vi "Plot_Channels_TF.vi"() -> (5 "Plug in titles":string[](array[string]), 7 "Plug in values":string[](array[string]))   [LabVIEW 2011]
uses:
  Controls/XY_Plot_Cluster.ctl
  Globals/Meas_global.vi
panel:
  out "Stats Array":string[][](array[string])
  in  "Run Spectra":bool=TRUE
  in  "Run Stats":bool=TRUE
  in  "Time delay":dbl
  in  "Save plot":bool
  in  "Save Plot":bool
  out "XY Graph 2":cluster{"Time (ms)":dbl[], "Eng Values":dbl[]}[](graph)
  out "Stats out":T1
  out "Size 2":i32
  out "Size 1":i32
  out "Size 0":i32
  in  "interp. method":i32(ring) items=["nearest", "linear", "spline", "cubic Hermite", "Lagrange"]
  in  "index 2":i32=3
  out "XY Graph":cluster{"Time (ms)":dbl[], "Eng Values":dbl[]}[](graph)
  in  "index 1":i32=1
  in  "index 0":i32
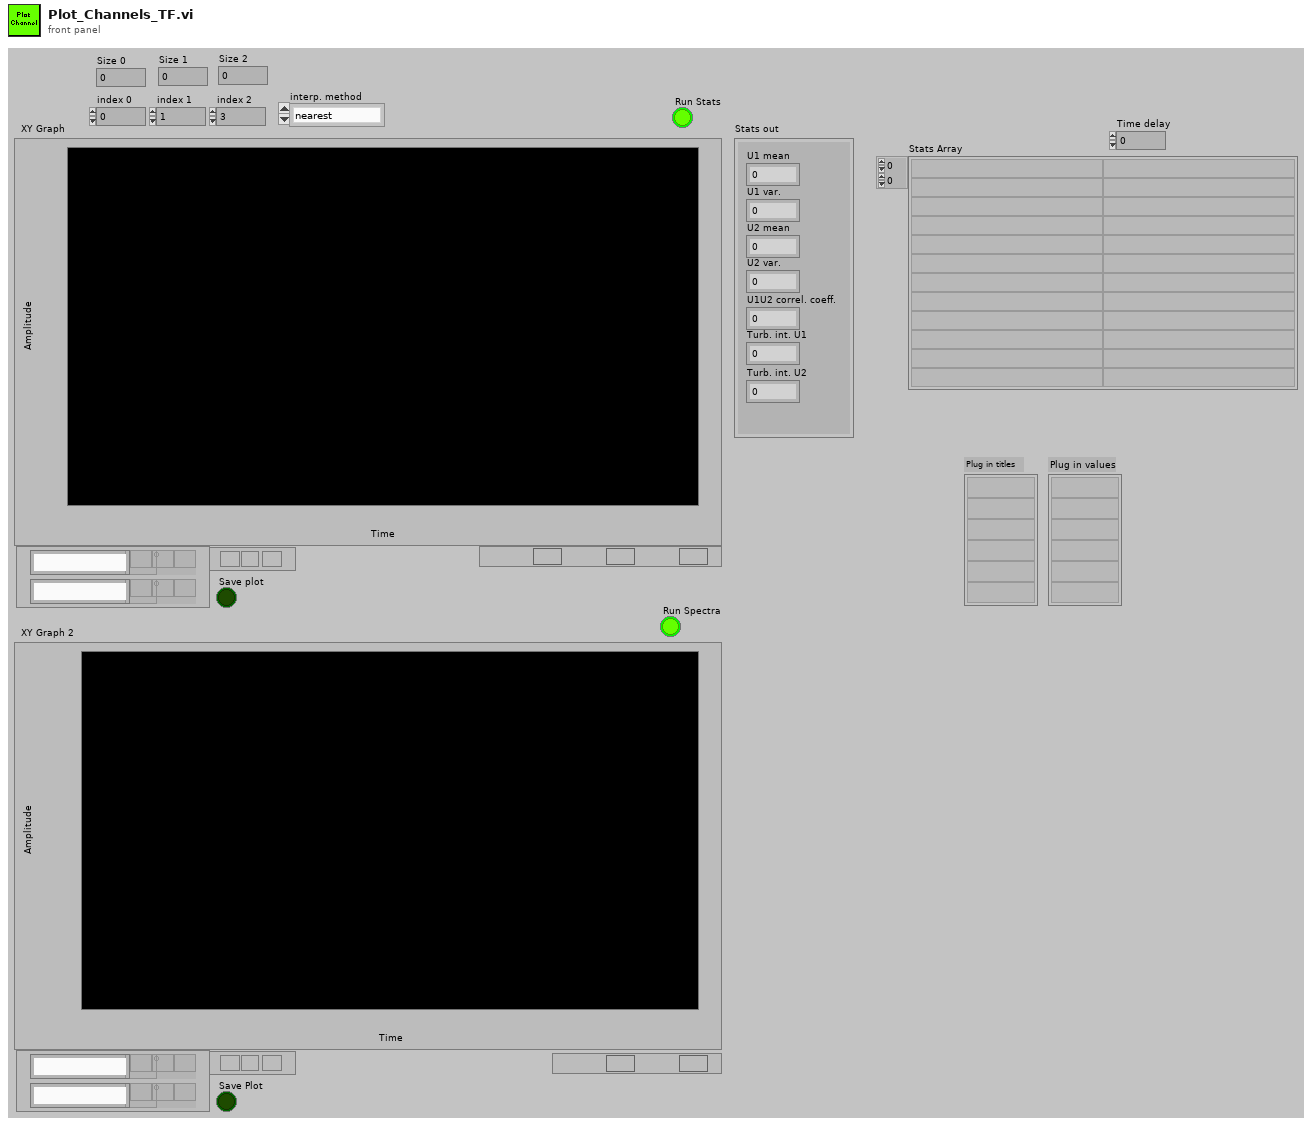
[diagram p1: front panel]
types:
  T1 = cluster{"U1 mean":dbl, "U1 var.":dbl, "U2 mean":dbl, "U2 var.":dbl, "U1U2 correl. coeff.":dbl, "Turb. int. U1":dbl, "Turb. int. U2":dbl}
  T2 = typedef "Analysis_info_cluster.ctl" = cluster{"Colour":u32, "Inst type":T3, "Inst name":string, "Symbol":string, "Code name":string, "Extra Info":string, "Inst Array":T4, "Index":i32, "Voltage Index":i32, "Extra Titles":string[], "Extra Values":string[], "Eng Values":dbl[], "Time (ms)":dbl[], "TT / Voltage":dbl[], "U":dbl, "u^2":dbl, "u^3":dbl, "u^4":dbl, "Skew_u":dbl, "Kurt_u":dbl, "Mean % Err":dbl, "% u'/U":dbl, "X":dbl, "Y":dbl, "Z":dbl}
  T3 = typedef "Inst_type.ctl" = enum16{"Propeller anemometer", "Raw voltage", "Pressure Transducer", "Pitot-static tube", "Preston tube", "Hot wire", "Cross wire 1", "Cross wire 2", "Generic Linear", "Generic Polynomial", "Generic BackPoly", "Fast FID", "Thermocouple", "Cold wire", "Pulsed Wire", "LDA Vel", "LDA Tran time", "LDA Arr time"}
  T4 = typedef "Instrument_Array.ctl" = enum16{"PWA", "LDA", "Analogue"}
  T5 = typedef "XY_Plot_Cluster.ctl" = cluster{"First Name":string, "Second Name":string, "X axis name":string, "Y axis name":string, "X array":dbl[], "Y array":dbl[]}
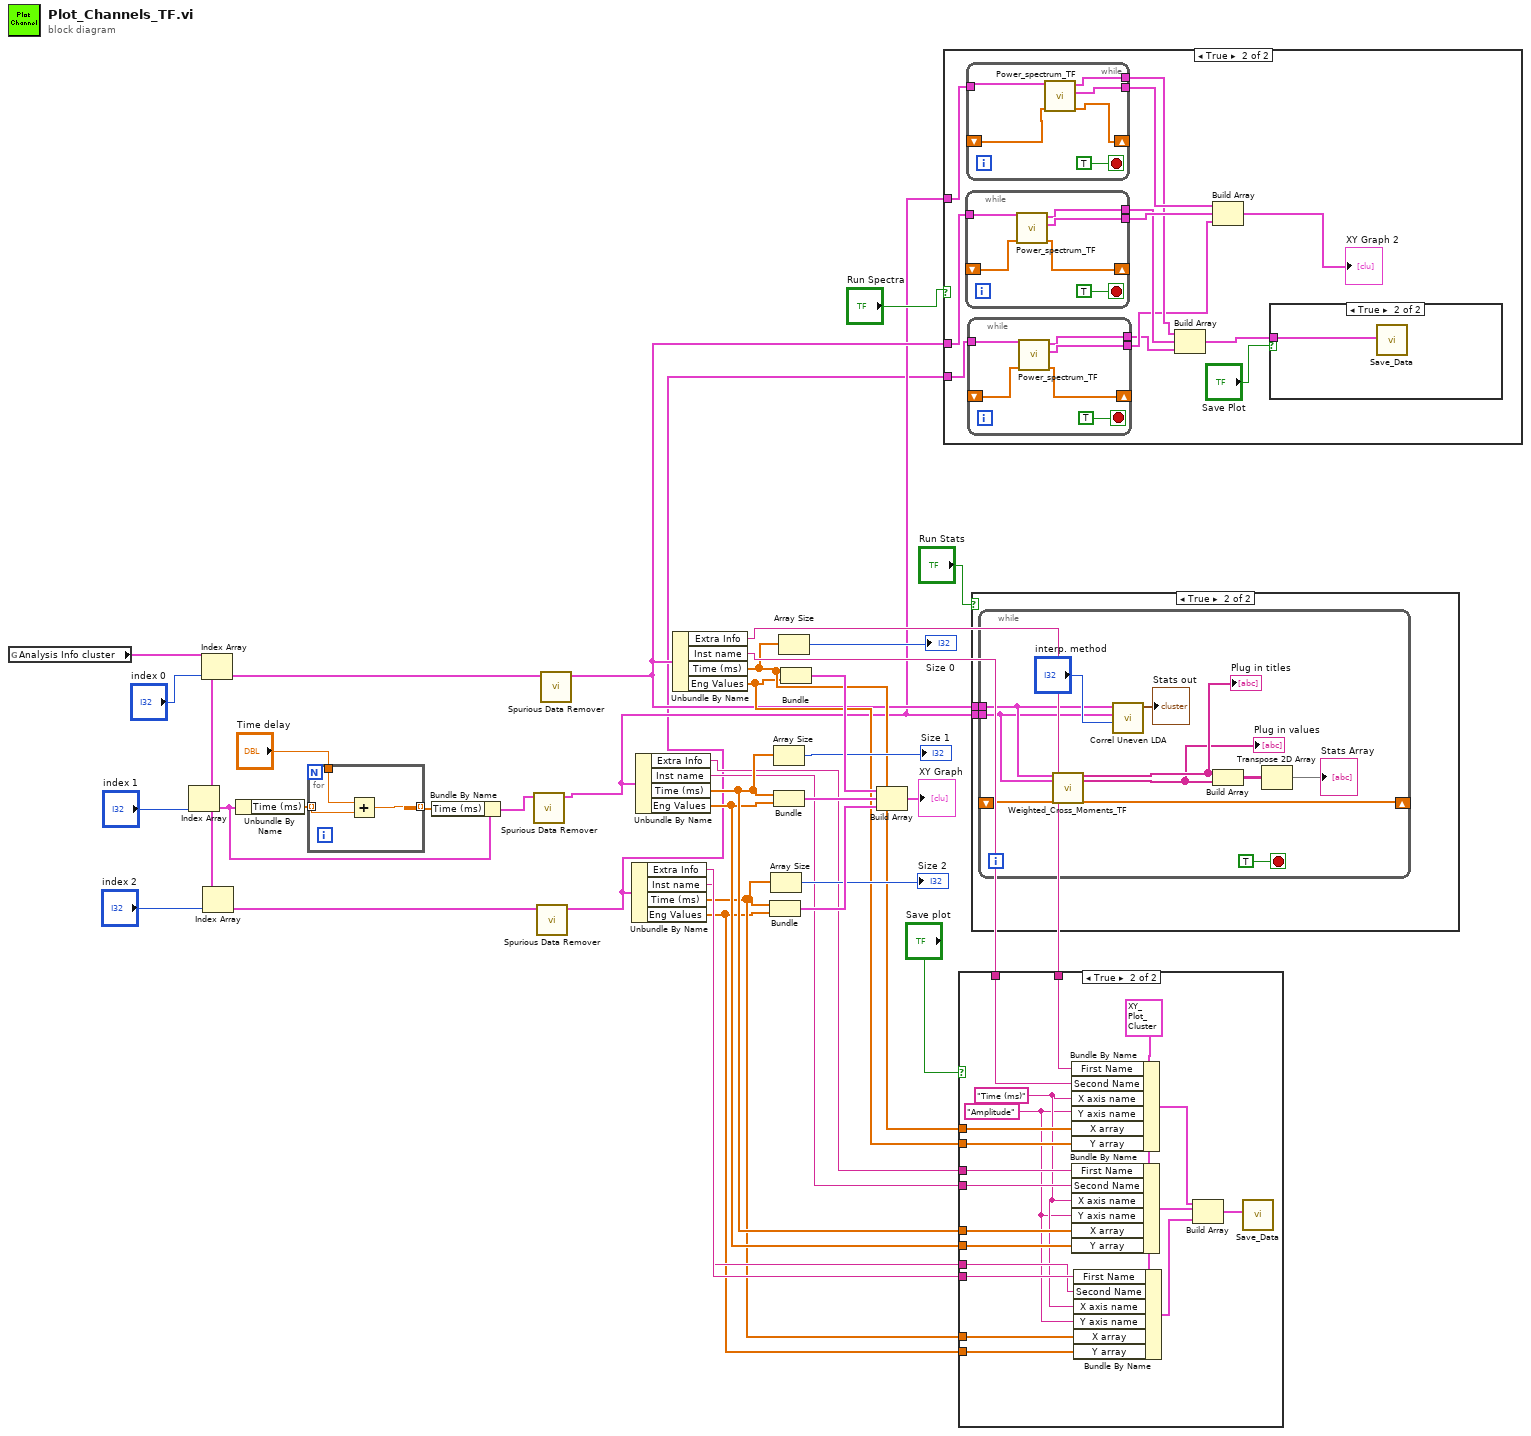
[diagram p0: block diagram]
diagram:
  n1 = global read "Meas_global.vi" "Analysis Info cluster"() -> (w12:T2[])
  n2 = Index Array(array=w12, index="index 1") -> (element=w6:T2)
  n3 = Index Array(array=w12, index="index 0") -> (element=w8:T2)
  n4 = Index Array(array=w12, index="index 2") -> (element=w27:T2)
  n5 = Unbundle By Name(w6) -> ("Time (ms)"=w11:dbl[])
  n6 = for {
    tunnel: w11 -> [w39] mode=indexing
    tunnel: [w38] -> w10 mode=indexing
    tunnel: "Time delay" -> [w37]
    n7 = Add(x=w37, y=w39) -> (x+y=w38:dbl)
  }
  n8 = Bundle By Name(cluster=w6, "Time (ms)"=w10) -> (w9:T2)
  n9 = call "Spurious Data Remover.vi"("Cluster 1"=w9) -> ("Cluster 1 Spurious points removed"=w2:T2)  [unwired: 10 in]
  n10 = call "Spurious Data Remover.vi"("Cluster 1"=w27) -> ("Cluster 1 Spurious points removed"=w1:T2)  [unwired: 10 in]
  n11 = call "Spurious Data Remover.vi"("Cluster 1"=w8) -> ("Cluster 1 Spurious points removed"=w3:T2)  [unwired: 10 in]
  n12 = Unbundle By Name(w1) -> ("Extra Info"=w16:string, "Inst name"=w15:string, "Time (ms)"=w14:dbl[], "Eng Values"=w13:dbl[])
  n13 = Unbundle By Name(w2) -> ("Extra Info"=w17:string, "Inst name"=w18:string, "Time (ms)"=w20:dbl[], "Eng Values"=w19:dbl[])
  n14 = Unbundle By Name(w3) -> ("Extra Info"=w25:string, "Inst name"=w24:string, "Time (ms)"=w23:dbl[], "Eng Values"=w22:dbl[])
  n15 = Bundle("Time (ms)"=w14, "Eng Values"=w13) -> (w31:cluster{"Time (ms)":dbl[], "Eng Values":dbl[]})  [unwired: 1 in]
  n16 = Array Size(array=w14) -> (size(s)=→"Size 2":i32)
  n17 = Array Size(array=w20) -> (size(s)=→"Size 1":i32)
  n18 = Bundle("Time (ms)"=w20, "Eng Values"=w19) -> (w34:cluster{"Time (ms)":dbl[], "Eng Values":dbl[]})  [unwired: 1 in]
  n19 = Array Size(array=w23) -> (size(s)=→"Size 0":i32)
  n20 = Bundle("Time (ms)"=w23, "Eng Values"=w22) -> (w33:cluster{"Time (ms)":dbl[], "Eng Values":dbl[]})  [unwired: 1 in]
  n21 = Build Array(w33, w34, w31) -> (→"XY Graph":cluster{"Time (ms)":dbl[], "Eng Values":dbl[]}[])
  n22 = case shown="True" "Run Spectra" {
    tunnel: w3 -> [_ w43]
    tunnel: w2 -> [_ w51]
    tunnel: w1 -> [_ w42]
    frame False {
    }
    frame True {
      n23 = while {
        tunnel: w43 -> [w69]
        shift-right: [w67] -> _
        shift-left: _ -> [w68]
        tunnel: [w66] -> w50
        tunnel: [w65] -> w47
        stop <- TRUE stop-if-true
        n24 = call "Power_spectrum_TF.vi"("Spectrum input array"=w68, "Cluster 1"=w69) -> ("Spectrum output array"=w67:dbl[], "XY Graph"=w66:cluster{dbl[], dbl[]}, "XY Plot Cluster"=w65:T5)  [unwired: 4 in]
      }
      n25 = while {
        tunnel: w51 -> [w63]
        shift-right: [w60] -> _
        shift-left: _ -> [w62]
        tunnel: [w61] -> w49
        tunnel: [w59] -> w46
        stop <- TRUE stop-if-true
        n26 = call "Power_spectrum_TF.vi"("Spectrum input array"=w62, "Cluster 1"=w63) -> ("Spectrum output array"=w60:dbl[], "XY Graph"=w61:cluster{dbl[], dbl[]}, "XY Plot Cluster"=w59:T5)  [unwired: 4 in]
      }
      n27 = while {
        tunnel: w42 -> [w56]
        shift-right: [w54] -> _
        shift-left: _ -> [w55]
        tunnel: [w53] -> w41
        tunnel: [w52] -> w40
        stop <- TRUE stop-if-true
        n28 = call "Power_spectrum_TF.vi"("Spectrum input array"=w55, "Cluster 1"=w56) -> ("Spectrum output array"=w54:dbl[], "XY Graph"=w53:cluster{dbl[], dbl[]}, "XY Plot Cluster"=w52:T5)  [unwired: 4 in]
      }
      n29 = Build Array(w46, w47, w40) -> (w45:T5[])
      n30 = Build Array(w49, w50, w41) -> (→"XY Graph 2":cluster{dbl[], dbl[]}[])
      n31 = case shown="True" "Save Plot" {
        tunnel: w45 -> [_ w58]
        frame False {
        }
        frame True {
          n32 = call "Save_Data.vi"("appended array"=w58) -> ()  [unwired: 11 in]
        }
      }
    }
  }
  n33 = case shown="True" "Save plot" {
    tunnel: w25 -> [_ w89]
    tunnel: w24 -> [_ w88]
    tunnel: w23 -> [_ w87]
    tunnel: w22 -> [_ w86]
    tunnel: w20 -> [_ w80]
    tunnel: w19 -> [_ w79]
    tunnel: w18 -> [_ w78]
    tunnel: w17 -> [_ w77]
    tunnel: w16 -> [_ w76]
    tunnel: w15 -> [_ w75]
    tunnel: w14 -> [_ w72]
    tunnel: w13 -> [_ w71]
    frame False {
    }
    frame True {
      w73 = "Amplitude" ("Y axis name")
      w74 = "Time (ms)" ("X axis name")
      w85 = T5 {"First Name"="Green", "Second Name"="LDA (U1)", "X axis name"="Green", "Y axis name"="Green", "X array"=array[8192 elements], "Y array"=array[8192 elements]} ("XY Plot cluster")
      n34 = Bundle By Name(cluster=w85, "First Name"=w89, "Second Name"=w88, "X axis name"=w74, "Y axis name"=w73, "X array"=w87, "Y array"=w86) -> (w84:T5)
      n35 = Bundle By Name(cluster=w85, "First Name"=w77, "Second Name"=w78, "X axis name"=w74, "Y axis name"=w73, "X array"=w80, "Y array"=w79) -> (w83:T5)
      n36 = Bundle By Name(cluster=w85, "First Name"=w76, "Second Name"=w75, "X axis name"=w74, "Y axis name"=w73, "X array"=w72, "Y array"=w71) -> (w82:T5)
      n37 = Build Array(w84, w83, w82) -> (w81:T5[])
      n38 = call "Save_Data.vi"("appended array"=w81) -> ()  [unwired: 11 in]
    }
  }
  n39 = case shown="True" "Run Stats" {
    tunnel: w3 -> [_ w91]
    tunnel: w2 -> [_ w90]
    frame False {
    }
    frame True {
      n40 = while {
        tunnel: w91 -> [w100]
        tunnel: w90 -> [w99]
        shift-right: [w98] -> _
        shift-left: _ -> [w97]
        stop <- TRUE stop-if-true
        n41 = call "Weighted_Cross_Moments_TF.vi"("Cluster 1"=w100, "Cluster 2"=w99, "Shift in"=w97) -> ("Headers"=w93:string[], "Results"=w92:string[], "Shift out"=w98:dbl[])  [unwired: 14 in]
        "Plug in titles" <- w93
        "Plug in values" <- w92
        n42 = call "Correl Uneven LDA.vi"("interp. method"="interp. method", "Cluster 2"=w99, "Cluster 1"=w100) -> ("Stats out"=→"Stats out":T1)  [unwired: 8 in]
        n43 = Build Array(w93, w92) -> (w95:string[][])
        n44 = Transpose 2D Array(2D array=w95) -> (transposed array=→"Stats Array":string[][])
      }
    }
  }
